vi "Read Waveform.vi"(0 "VISA resource name":refnum<visa-resource-name>, 1 "End Point (1000)":u32=1000 max=4000000 step=1, 2 "Start Point (0)":u32 max=4000000 step=1, 5 "Select Trace (1)":u16=1 min=1 max=32 step=1, 11 "error in (no error)":errorcluster) -> (4 "VISA resource name out":refnum<visa-resource-name>, 6 "Waveform Data":string, 15 "error out":errorcluster)   [LabVIEW 2013, in "Yokogawa PZ4000.lvlib"]
doc: "This VI reads the Waveform Data from the PZ4000 series.\nWaveform Read Function is Send Command and Read Waveform Data."
uses:
  <instrlib>/Yokogawa PZ4000/Yokogawa PZ4000.lvlib
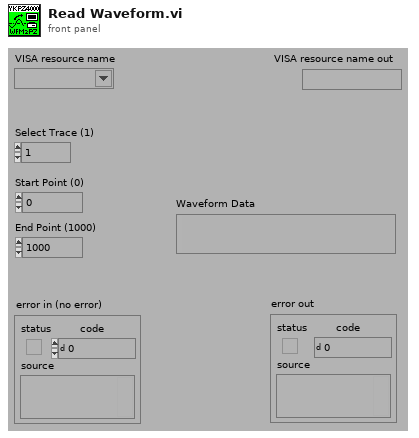
[diagram p1: front panel]
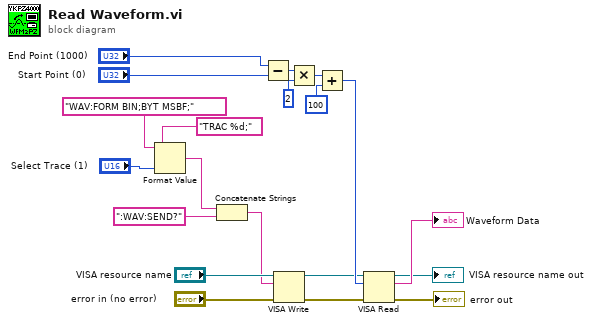
[diagram p0: block diagram]
diagram:
  n1 = Format Value(string ("")="WAV:FORM BIN;BYT MSBF;", format string="TRAC %d;", value (0)="Select Trace (1)") -> (output string=w3:string)
  n2 = Concatenate Strings(w3, ":WAV:SEND?") -> (w4:string)
  n3 = Subtract(x="End Point (1000)", y="Start Point (0)") -> (x-y=w20:u32)
  n4 = VISA Write(VISA resource name="VISA resource name", write buffer=w4, error in (no error)="error in (no error)") -> (VISA resource name out=w12:refnum<visa-resource-name>, error out=w14:errorcluster)  [unwired: 1 out]
  n5 = Multiply(x=w20, y=u32 2) -> (x*y=w17:u32)
  n6 = Add(x=w17, y=u32 100) -> (x+y=w13:u32)
  n7 = VISA Read(VISA resource name=w12, byte count=w13, error in (no error)=w14) -> (VISA resource name out=→"VISA resource name out":refnum<visa-resource-name>, read buffer=→"Waveform Data":string, error out=→"error out":errorcluster)  [unwired: 1 out]
